vi "Source using Agilent and Keithley.vi"() -> ()   [LabVIEW 2021]
doc: "This example shows how to configure a measurement and take a reading."
uses:
  <instrlib>/Keithley 24XX/Public/Data/Read (Single Point).vi
  <instrlib>/Keithley 24XX/Keithley 24XX.lvlib
  <instrlib>/Agilent N6700 Series/Agilent N6700 Series.lvlib
panel:
  in  "Agilent SMU":refnum<visa-resource-name>
  in  "Channel Name":string="1"
  in  "Voltage Range":dbl=10.0 format="%^.3e"
  in  "Voltage Level":dbl=5.0 format="%^.3e"
  out "Agilent Voltage Measurement":dbl format="%^.3e"
  out "Keithly Resistance":sgl
  out "Keithly  Current":sgl
  out "Keithly Voltage":sgl
  in  "error in":errorcluster
  out "error out":errorcluster
  in  "Source Mode":u16(ring) items=["Voltage", "Current"]
  in  "Compliance  Level (0.1)":dbl=0.1
  in  "Output Level (0)":dbl
  in  "Resistance Manual Range":dbl=1.0
  in  "Current Manual Range":dbl=1.0
  in  "Voltage Manual Range":dbl=1.0
  in  "Keithley SMU":refnum<visa-resource-name>
  # "(c) 2006 National Instruments.  ALL RIGHTS RESERVED."
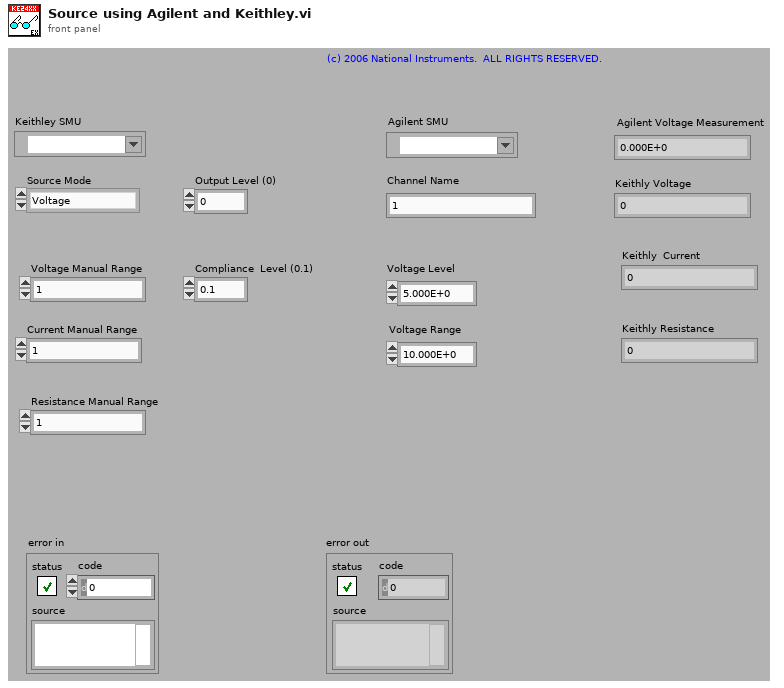
[diagram p1: front panel]
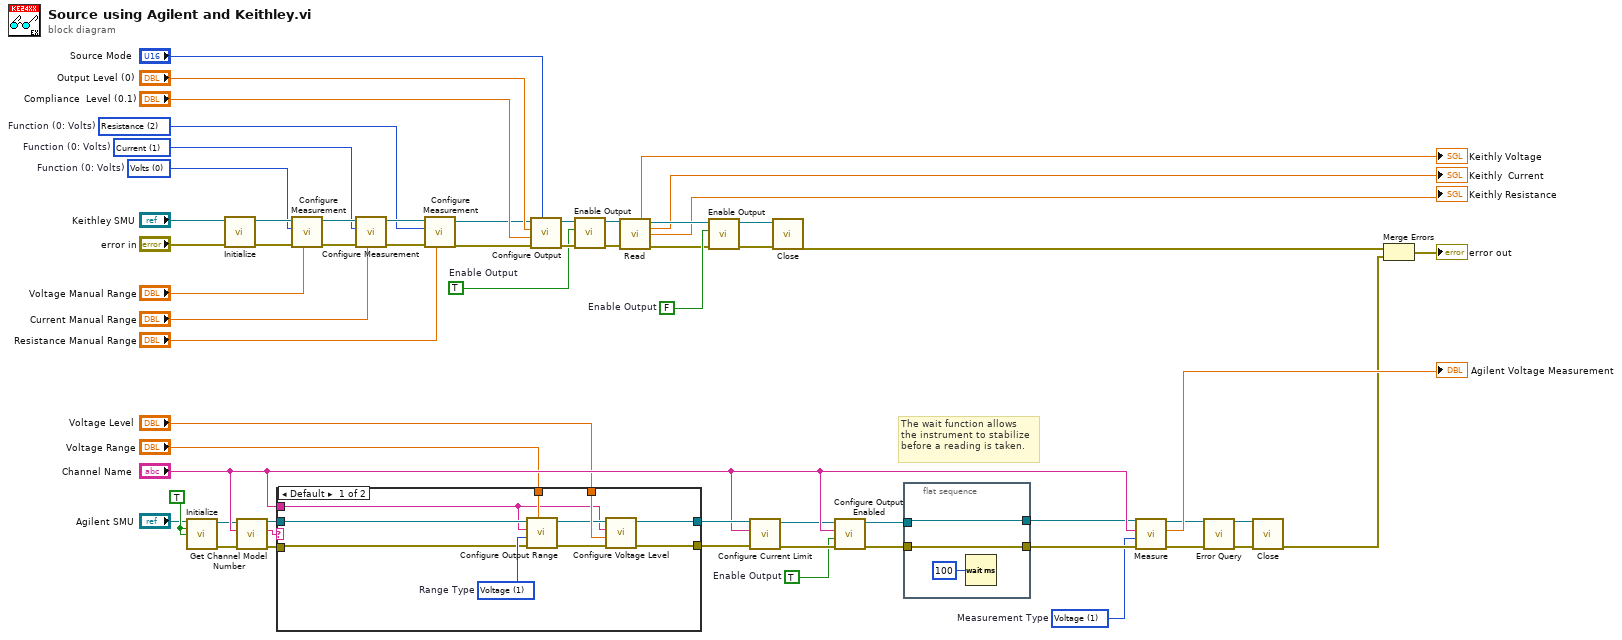
[diagram p0: block diagram]
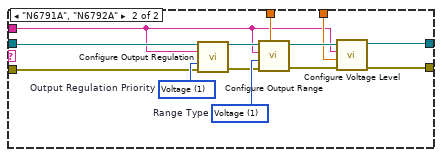
[diagram p2: hidden frame]
diagram:
  w12 = TRUE ("Reset? (T: Yes)")
  w11 = 1 items=["Voltage"=1, "Current"=0]  # Measurement Type
  w10 = TRUE  # Enable Output
  w36 = TRUE  # Enable Output
  w47 = FALSE  # Enable Output
  w51 = u16 2 items=["Volts", "Current", "Resistance"]  # Function (0: Volts)
  w52 = u16 1 items=["Volts", "Current", "Resistance"]  # Function (0: Volts)
  w53 = u16 0 items=["Volts", "Current", "Resistance"]  # Function (0: Volts)
  # "The wait function allows \nthe instrument to stabilize\nbefore a reading is taken."
  n1 = call <instrlib>:"Initialize.vi"("VISA resource name"="Agilent SMU", "ID Query? (T: Yes)"=w12, "Reset? (T: Yes)"=w12) -> ("VISA resource name out"=w19:refnum<visa-resource-name>, "error out"=w20:errorcluster)  [unwired: 11 in]
  n2 = call <instrlib>:"Initialize.vi"("error in (no error)"="error in", "VISA resource name"="Keithley SMU") -> ("error out"=w58:errorcluster, "VISA resource name out"=w59:refnum<visa-resource-name>)  [unwired: 8 in]
  n3 = call <instrlib>:"Get Channel Model Number.vi"("error in (no error)"=w20, "Channel Name (1)"="Channel Name", "VISA resource name"=w19) -> ("error out"=w22:errorcluster, "Model Number"=w23:string, "VISA resource name out"=w21:refnum<visa-resource-name>)  [unwired: 6 in]
  n4 = case shown="Default" w23 {
    tunnel: "Voltage Range" -> [w67 w83]
    tunnel: "Channel Name" -> [w61 w73]
    tunnel: w21 -> [w69 w78]
    tunnel: w22 -> [w68 w77]
    tunnel: "Voltage Level" -> [w65 w74]
    tunnel: [w63 w71] -> w26
    tunnel: [w62 w72] -> w27
    frame Default {
      w70 = 1 items=["Voltage"=1, "Current"=0]  # Range Type
      n5 = call <instrlib>:"Configure Output Range.vi"("Range (0.0)"=w67, "error in (no error)"=w68, "Range Type (1: Voltage)"=w70, "Channel Name (1)"=w61, "VISA resource name"=w69) -> ("error out"=w66:errorcluster, "VISA resource name out"=w64:refnum<visa-resource-name>)  [unwired: 5 in]
      n6 = call <instrlib>:"Configure Voltage Level.vi"("error in (no error)"=w66, "Level  (0.0 volts)"=w65, "Channel Name (1)"=w61, "VISA resource name"=w64) -> ("error out"=w63:errorcluster, "VISA resource name out"=w62:refnum<visa-resource-name>)  [unwired: 6 in]
    }
    frame "N6791A", "N6792A" {
      w79 = 1 items=["Voltage"=1, "Current"=0]  # Output Regulation Priority
      w82 = 1 items=["Voltage"=1, "Current"=0]  # Range Type
      n7 = call <instrlib>:"Configure Output Regulation.vi"("VISA resource name"=w78, "Channel Name (1)"=w73, "Output Regulation Priority (1: Voltage)"=w79, "error in (no error)"=w77) -> ("VISA resource name out"=w81:refnum<visa-resource-name>, "error out"=w80:errorcluster)  [unwired: 10 in]
      n8 = call <instrlib>:"Configure Output Range.vi"("Range (0.0)"=w83, "error in (no error)"=w80, "Range Type (1: Voltage)"=w82, "Channel Name (1)"=w73, "VISA resource name"=w81) -> ("error out"=w75:errorcluster, "VISA resource name out"=w76:refnum<visa-resource-name>)  [unwired: 5 in]
      n9 = call <instrlib>:"Configure Voltage Level.vi"("error in (no error)"=w75, "Level  (0.0 volts)"=w74, "Channel Name (1)"=w73, "VISA resource name"=w76) -> ("error out"=w71:errorcluster, "VISA resource name out"=w72:refnum<visa-resource-name>)  [unwired: 6 in]
    }
  }
  n10 = call <instrlib>:"Configure Measurement.vi"("Manual Range (1.0)"="Voltage Manual Range", "error in (no error)"=w58, "Function (0: Volts)"=w53, "VISA resource name"=w59) -> ("error out"=w56:errorcluster, "VISA resource name out"=w57:refnum<visa-resource-name>)  [unwired: 6 in]
  n11 = call <instrlib>:"Configure Measurement.vi"("Manual Range (1.0)"="Current Manual Range", "error in (no error)"=w56, "Function (0: Volts)"=w52, "VISA resource name"=w57) -> ("error out"=w55:errorcluster, "VISA resource name out"=w54:refnum<visa-resource-name>)  [unwired: 6 in]
  n12 = call <instrlib>:"Configure Measurement.vi"("Manual Range (1.0)"="Resistance Manual Range", "error in (no error)"=w55, "Function (0: Volts)"=w51, "VISA resource name"=w54) -> ("error out"=w35:errorcluster, "VISA resource name out"=w34:refnum<visa-resource-name>)  [unwired: 6 in]
  n13 = call <instrlib>:"Configure Output.vi"("Source Mode  (0: Voltage)"="Source Mode", "error in (no error)"=w35, "Compliance  Level (0.1)"="Compliance  Level (0.1)", "Output Level (0)"="Output Level (0)", "VISA resource name"=w34) -> ("error out"=w37:errorcluster, "VISA resource name out"=w38:refnum<visa-resource-name>)  [unwired: 5 in]
  n14 = call <instrlib>:"Enable Output.vi"("error in (no error)"=w37, "Enable Output (T: Enable)"=w36, "VISA resource name"=w38) -> ("error out"=w40:errorcluster, "VISA resource name out"=w39:refnum<visa-resource-name>)  [unwired: 7 in]
  n15 = call-poly <instrlib>:"Read.vi"("VISA resource name"=w39, "error in (no error)"=w40) -> ("Voltage"=→"Keithly Voltage":sgl, "VISA resource name out"=w41:refnum<visa-resource-name>, "Current"=→"Keithly  Current":sgl, "Resistance"=→"Keithly Resistance":sgl, "error out"=w42:errorcluster)  [unwired: 7 in, 2 out]
  n16 = call <instrlib>:"Enable Output.vi"("error in (no error)"=w42, "Enable Output (T: Enable)"=w47, "VISA resource name"=w41) -> ("error out"=w43:errorcluster, "VISA resource name out"=w44:refnum<visa-resource-name>)  [unwired: 7 in]
  n17 = call <instrlib>:"Configure Current Limit.vi"("error in (no error)"=w26, "Channel Name (1)"="Channel Name", "VISA resource name"=w27) -> ("error out"=w13:errorcluster, "VISA resource name out"=w14:refnum<visa-resource-name>)  [unwired: 7 in]
  n18 = call <instrlib>:"Close.vi"("error in (no error)"=w43, "VISA resource name"=w44) -> ("error out"=w32:errorcluster)  [unwired: 9 in]
  n19 = call <instrlib>:"Configure Output Enabled.vi"("error in (no error)"=w13, "Enable Output (False)"=w10, "Channel Name (1)"="Channel Name", "VISA resource name"=w14) -> ("error out"=w18:errorcluster, "VISA resource name out"=w15:refnum<visa-resource-name>)  [unwired: 6 in]
  n20 = flat-sequence {
    tunnel: w15 -> [w86]
    tunnel: [w86] -> w16
    tunnel: [w84] -> w17
    tunnel: w18 -> [w84]
    frame #0 {
      n21 = Wait (ms)(milliseconds to wait=u32 100) -> ()  [unwired: 1 out]
    }
  }
  n22 = call <instrlib>:"Measure.vi"("error in (no error)"=w17, "Measurement Type (1: Voltage)"=w11, "Channel Name (1)"="Channel Name", "VISA resource name"=w16) -> ("error out"=w3:errorcluster, "Measurement"=→"Agilent Voltage Measurement":dbl, "VISA resource name out"=w6:refnum<visa-resource-name>)  [unwired: 5 in]
  n23 = call <instrlib>:"Error Query.vi"("VISA resource name"=w6, "error in (no error)"=w3) -> ("VISA resource name out"=w5:refnum<visa-resource-name>, "error out"=w4:errorcluster)  [unwired: 10 in, 2 out]
  n24 = call <instrlib>:"Close.vi"("VISA resource name"=w5, "error in (no error)"=w4) -> ("error out"=w1:errorcluster)  [unwired: 13 in]
  n25 = Merge Errors(w32, w1) -> (→"error out":errorcluster)
